vi "Processing module error handling.vi"(8 "error in (no error)":errorcluster, 11 "Imaging Protocol":T1) -> ()   [LabVIEW 2020]
uses:
  Typedefs/Imaging Protocols enum.ctl
  Typedefs/Top level VI states.ctl
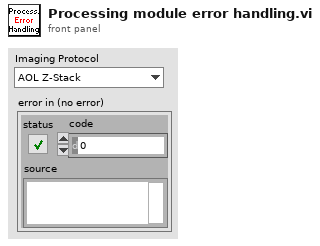
[diagram p1: front panel]
types:
  T1 = typedef "Imaging Protocols enum.ctl" = enum16{"AOL Z-Stack", "Motor Z Stack", "Functional Acquisition", "Single Plane Acquisition", "Volume Acquisition", "Live Imaging", "Live Plane Imaging", "Live Volume Imaging"}
  T2 = typedef "Top level VI states.ctl" = enum16{"None", "Initialise UI", "<STACK PROTOCOL STATES>", "AOL Zstack-START", "AOL Zstack-STOP", "Motor Zstack-START", "Motor Zstack-STOP", "<ACQUISITION PROTOCOL STATES> ", "Functional Acquisition-START", "Functional Acquisition-STOP", "Single Plane Acquisition-START", "Single Plane Acquisition-STOP", "Volume Acquisition-START", "Volume Acquisition-STOP", "<LIVE IMAGING PROTOCOL STATES>", "Live Imaging-START", "Live Imaging-STOP", "Live Plane Imaging-START", "Live Plane Imaging-STOP", "Live Volume Imaging-START", "Live Volume Imaging-STOP", "<MOVEMENT CORRECTION PROTOCOL STATES>", "EXIT"}
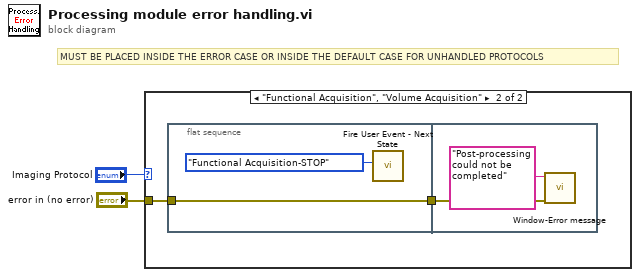
[diagram p0: block diagram]
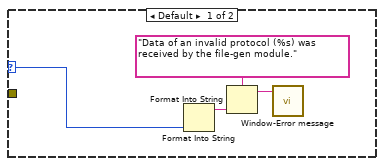
[diagram p2: hidden frame]
diagram:
  # "MUST BE PLACED INSIDE THE ERROR CASE OR INSIDE THE DEFAULT CASE FOR UNHANDLED PROTOCOLS"
  n1 = case shown="\"Functional Acquisition\", \"Volume Acquisition\"" "Imaging Protocol" {
    selector: "Imaging Protocol" -> [w3 _]
    tunnel: "error in (no error)" -> [_ w7]
    frame Default {
      n2 = Format Into String(w3) -> (resulting string=w5:string)  [unwired: 3 in, 1 out]
      n3 = Format Into String(format string="Data of an invalid protocol (%s) was received by the file-gen module." ("Error Source"), w5) -> (resulting string=w4:string)  [unwired: 2 in, 1 out]
      n4 = call "Window-Error message.vi"("Message"=w4) -> ()  [unwired: 10 in, 1 out]
    }
    frame "Functional Acquisition", "Volume Acquisition" {
      n5 = flat-sequence {
        tunnel: w7 -> [w9]
        tunnel: [w9] -> w8
        tunnel: w8 -> [w11]
        frame #0 {
          n6 = call "Fire User Event - Next State.vi"("\"UI Handler loop\" case to execute"=Top_level_VI_states."Functional Acquisition-STOP" ("event data / imaging mode")) -> ()  [unwired: 10 in, 1 out]
        }
        frame #1 {
          n7 = call "Window-Error message.vi"("error in (no error)"=w11, "Message"="Post-processing could not be completed") -> ()  [unwired: 9 in, 1 out]
        }
      }
    }
  }
